vi "Get Custom Device Session IP Address.vi"(8 "error in (no error)":errorcluster, 11 "Item Ref in":T1 format="%.0x") -> (0 "error out":errorcluster, 2 "IP Address":string, 3 "Item Ref out":T1 format="%.0x")   [LabVIEW 2015, in "Shared Variable Custom Device.lvlib"]
uses:
  Shared Variable Custom Device.lvlib
  <vilib>/NI Veristand/Custom Device API/Custom Device Item Ref.ctl
  <vilib>/NI Veristand/Custom Device Tools/Custom Device Utility Library/Search Direction.ctl
  Shared Variable GUID Lookup.vi
  <vilib>/NI Veristand/Custom Device Tools/Custom Device Utility Library/NI VeriStand - Search for Item by GUID.vi
  <vilib>/NI Veristand/Custom Device Tools/Custom Device Utility Library/Custom Device Utility Library.lvlib
  <vilib>/NI Veristand/Custom Device API/Custom Device API.lvlib
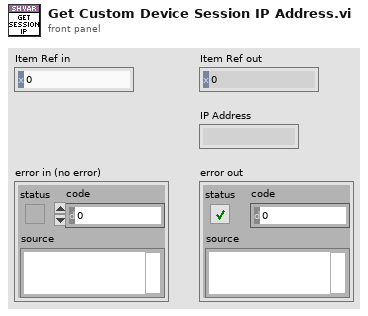
[diagram p1: front panel]
types:
  T1 = typedef "Custom Device API.lvlib/Custom Device Item Ref.ctl" = u64
  T2 = typedef "Custom Device Utility Library.lvlib/Search Direction.ctl" = enum16{"Down", "Up"}
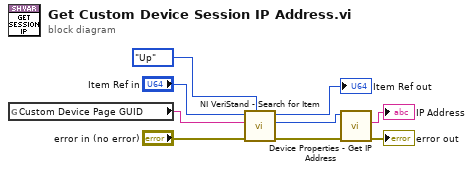
[diagram p0: block diagram]
diagram:
  n1 = global read "Shared Variable GUID Lookup.vi" "Custom Device Page GUID"() -> (w8:string)
  n2 = call-poly <vilib>:"NI VeriStand - Search for Item.vi"("Direction (Down)"=Search_Direction."Up", "error in"="error in (no error)", "Item GUID"=w8, "Section Ref in"="Item Ref in") -> ("error out"=w7:errorcluster, "Item Ref"=w6:T1, "Section Ref out"=→"Item Ref out":T1)  [unwired: 4 in, 1 out]
  n3 = call "Device Properties - Get IP Address.vi"("error in (no error)"=w7, "Device Ref in"=w6) -> ("error out"=→"error out":errorcluster, "IP Address"=→"IP Address":string)  [unwired: 7 in, 1 out]
